vi "DidInit.vi"(7 "Init?":bool, 8 "error in (no error)":errorcluster, 11 "ModuleAdmin":refnum<class "ModuleAdmin.lvclass">) -> (0 "error out":errorcluster)   [LabVIEW 2018, in "MyPlugins.lvlib"]
doc: "Sends a message from the module indicating that it successfully initialized."
uses:
  MyPlugins.lvlib
  <userlib>/NIST/ModuleAdminLib/ModuleAdmin/ModuleAdmin.lvclass
  PluginsShared/clDidInit.ctl
  PluginsShared/clEventType.ctl
  PluginsShared/PluginsShared.lvlib
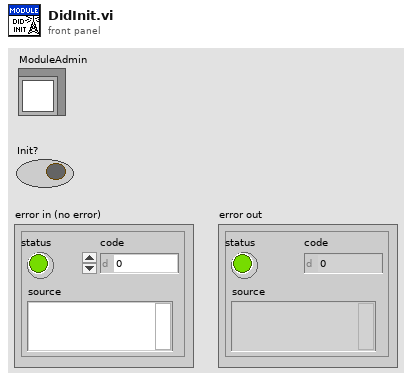
[diagram p1: front panel]
types:
  T1 = typedef "PluginsShared.lvlib/clEventType.ctl" = cluster{"ModuleID":i32, "Data":variant}
  T2 = typedef "PluginsShared.lvlib/clDidInit.ctl" = cluster{"Init?":bool, "ModuleAdmin":refnum<class "ModuleAdmin.lvclass">}
  T3 = typedef "PluginsShared.lvlib/clBroadcastEvents.ctl" = cluster{"DidInit":refnum<user-event>, "StatusUpdate":refnum<user-event>, "ErrorReport":refnum<user-event>, "DidStop":refnum<user-event>, "PathToINI":refnum<user-event>, "ReloadINIFiles":refnum<user-event>}
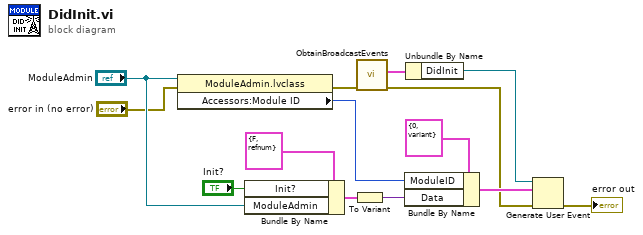
[diagram p0: block diagram]
diagram:
  n1 = property class="ModuleAdmin.lvclass"(reference="ModuleAdmin", error in="error in (no error)") -> (error out=w3:errorcluster, "Accessors:Module ID"=w5:i32)  [unwired: 1 out]
  n2 = Bundle By Name(cluster=T2 {"Init?"=FALSE, "ModuleAdmin"=refnum} ("clDidInit"), "Init?"="Init?", "ModuleAdmin"="ModuleAdmin") -> (w12:T2)
  n3 = To Variant(anything=w12) -> (Variant=w9:variant)
  n4 = call "ObtainBroadcastEvents.vi"("error in (no error)"=w3) -> ("error out"=w2:errorcluster, "clBroadcastEvents"=w13:T3)  [unwired: 9 in]
  n5 = Bundle By Name(cluster=T1 {"ModuleID"=0, "Data"=variant} ("clBroadcast"), "ModuleID"=w5, "Data"=w9) -> (w8:T1)
  n6 = Unbundle By Name(w13) -> ("DidInit"=w11:refnum<user-event>)
  n7 = Generate User Event(user event=w11, event data cluster=w8, error in=w2) -> (error out=→"error out":errorcluster)  [unwired: 1 in, 1 out]
